vi "FXP NIPLL_CostaLoop.vi"(8 "reset?":bool, 9 "norminal freq [U16.0]":fxp<+,16,0>, 10 "alpha [U16.0]":fxp<+,16,0>, 11 "x[I24.1]":fxp<+/-,24,1>) -> (0 "f":fxp<+/-,32,0> format="%.32g", 1 "z [I32.1]":fxp<+/-,32,1>, 2 "sin(z)":fxp<+/-,16,2> format="%.15g", 3 "cos(z)":fxp<+/-,16,2> format="%.15g")   [LabVIEW 2016]
uses:
  <vilib>/rvi/Emulation/niFpgaGetClockAttributes.vi
  <vilib>/rvi/Emulation/niFpgaSctlEmulationGetInTimedLoop.vi
  <vilib>/rvi/Emulation/niFpgaEmulationReportErrorSimple.vi
  <vilib>/rvi/Emulation/niFpgaCriticalErrorInLSC.vi
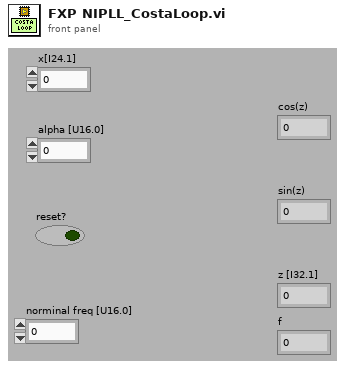
[diagram p1: front panel]
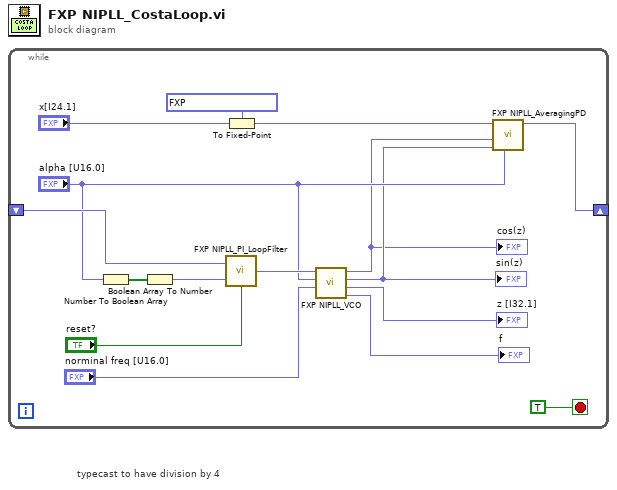
[diagram p0: block diagram]
diagram:
  # "typecast to have division by 4"
  n1 = while {
    shift-right: [w15] -> _
    shift-left: _ -> [w12]
    stop <- TRUE stop-if-true
    n2 = Number To Boolean Array(number="alpha [U16.0]") -> (Boolean array=w10:bool[])
    n3 = Boolean Array To Number(Boolean array=w10) -> (number=w9:fxp<+,16,-2>)
    n4 = call "FXP NIPLL_PI_LoopFilter.vi"("reset?"="reset?", "alpha [U16.-2]"=w9, "x [I16.2]"=w12) -> ("x+y [I48.17]"=w14:fxp<+/-,48,17>)
    n5 = To Fixed-Point(fixed-point type=fxp<+/-,16,1> 0.0 ("number"), number="x[I24.1]") -> (fixed-point=w1:fxp<+/-,16,1>)
    n6 = call "FXP NIPLL_VCO.vi"("nominal freq [U16.0]"="norminal freq [U16.0]", "Kv [U16.0]"="alpha [U16.0]", "v [I48.17]"=w14) -> ("f"=→"f":fxp<+/-,32,0>, "z [I32.1]"=→"z [I32.1]":fxp<+/-,32,1>, "sin(z) [I16.2]"=w5:fxp<+/-,16,2>, "cos(z) [I16.2]"=w4:fxp<+/-,16,2>)  [unwired: 5 in]
    "sin(z)" <- w5
    "cos(z)" <- w4
    n7 = call "FXP NIPLL_AveragingPD.vi"("alpha [U16.0]"="alpha [U16.0]", "sin(z) [I16.2]"=w5, "cos(z) [I16.2]"=w4, "x[I16.1]"=w1) -> ("psd_out"=w15:fxp<+/-,16,2>)  [unwired: 7 in]
  }
